vi "Bound_RO_R_R0I.vi"(6 "Bottom Right - Y":sgl, 9 "Right - X":sgl, 10 "Top Left - Y":sgl, 11 "Top  Left - x":sgl) -> (3 "ROI Descriptor":T1 {"Contours"."Type" items=["No Selection", "Point", "Line", "Rectangle", "Oval", "Polygon", "Freehand Region", "Annulus", "Unused2", "Unused3", "Broken Line", "Freehand Line", "Rotated Rectangle"]})   [LabVIEW 2015]
panel:
  in  "max Y (right)":sgl=220.0
  in  "max X (right)":sgl=320.0
  in  "min Y (left)":sgl
  in  "min X (left)":sgl
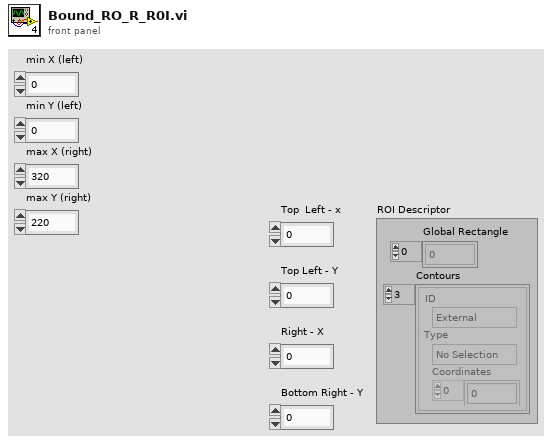
[diagram p1: front panel]
types:
  T1 = typedef "ROI Descriptor" = cluster{"Global Rectangle":i32[], "Contours":cluster{"ID":enum32{"External", "Internal"}, "Type":u32, "Coordinates":i32[]}[]}
  T2 = cluster{"min X (left)":sgl, "min Y (left)":sgl, "max X (right)":sgl, "max Y (right)":sgl, dbl}
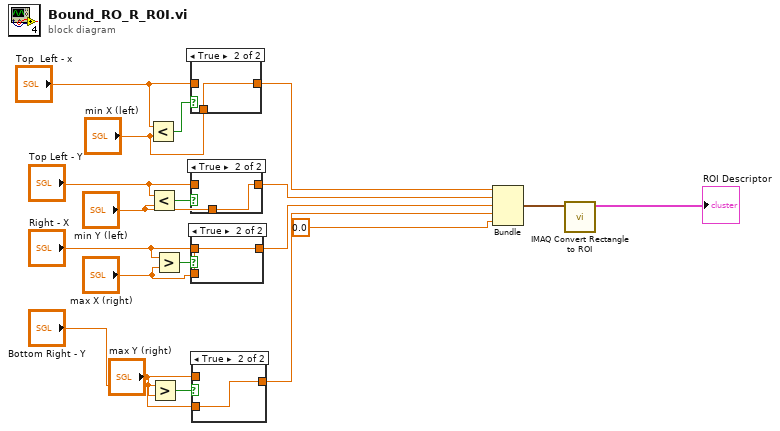
[diagram p0: block diagram]
diagram:
  n1 = Less?(x="Top  Left - x", y="min X (left)") -> (x < y?=w17:bool)
  n2 = Less?(x="Top Left - Y", y="min Y (left)") -> (x < y?=w16:bool)
  n3 = Greater?(x="Bottom Right - Y", y="max Y (right)") -> (0:w13:bool)
  n4 = Greater?(x="Right - X", y="max X (right)") -> (0:w15:bool)
  n5 = case shown="True" w17 {
    tunnel: [w20 w21] -> w9
    tunnel: "Top  Left - x" -> [w20 _]
    tunnel: "min X (left)" -> [_ w21]
    frame False {
    }
    frame True {
    }
  }
  n6 = case shown="True" w16 {
    tunnel: [w22 w23] -> w10
    tunnel: "Top Left - Y" -> [w22 _]
    tunnel: "min Y (left)" -> [_ w23]
    frame False {
    }
    frame True {
    }
  }
  n7 = case shown="True" w15 {
    tunnel: [w24 w25] -> w11
    tunnel: "Right - X" -> [w24 _]
    tunnel: "max X (right)" -> [_ w25]
    frame False {
    }
    frame True {
    }
  }
  n8 = case shown="True" w13 {
    tunnel: [w26 w27] -> w12
    tunnel: "Bottom Right - Y" -> [w26 _]
    tunnel: "max Y (right)" -> [_ w27]
    frame False {
    }
    frame True {
    }
  }
  n9 = Bundle("min X (left)"=w9, "min Y (left)"=w10, "max X (right)"=w11, "max Y (right)"=w12, 0.0) -> (w2:T2)  [unwired: 1 in]
  n10 = call "IMAQ Convert Rectangle to ROI"("Rectangle"=w2) -> ("ROI Descriptor"=→"ROI Descriptor":T1)  [unwired: 8 in, 1 out]
